vi "Shooting Boost.vi"(11 "Duration":dbl) -> (3 "Boost PWM":bool)   [LabVIEW 2016]
uses:
  Robot Global Data.vi
panel:
  # "Controls the duration of the forced PWM value when a ball is detected\nIf Zero, disable logic. Counterpart logic is located in Periodic Tasks"
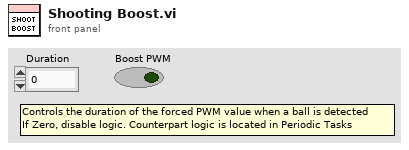
[diagram p1: front panel]
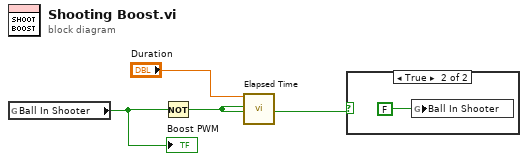
[diagram p0: block diagram]
diagram:
  n1 = global read "Robot Global Data.vi" "Ball In Shooter"() -> (w4:bool)
  "Boost PWM" <- w4
  n2 = Not(x=w4) -> (.not. x?=w2:bool)
  n3 = call "Elapsed Time"("Time Target (s)"="Duration", "Reset"=w2, "Auto Reset"=w2) -> ("Time has Elapsed"=w1:bool)  [unwired: 9 in, 7 out]
  n4 = case shown="True" w1 {
    frame False {
    }
    frame True {
      n5 = global write "Robot Global Data.vi" "Ball In Shooter"(FALSE) -> ()
    }
  }
